vi "Scroll Home.vi"(8 "error in":errorcluster, 10 "Tab Control":T1(ring), 11 "Report Viewer in":refnum<class "Report Viewer.lvclass">) -> (0 "error out":errorcluster, 3 "Report Viewer out":refnum<class "Report Viewer.lvclass">)   [LabVIEW 2019, in "Report Viewer.lvlib" / "Report Viewer.lvclass"]
uses:
  Library/Report Viewer.lvclass
  Library/Report Viewer.lvclass/Report Viewer.ctl
  <vilib>/Utility/miscctls.llb/LVRowAndColumnUnsignedTypeDef.ctl
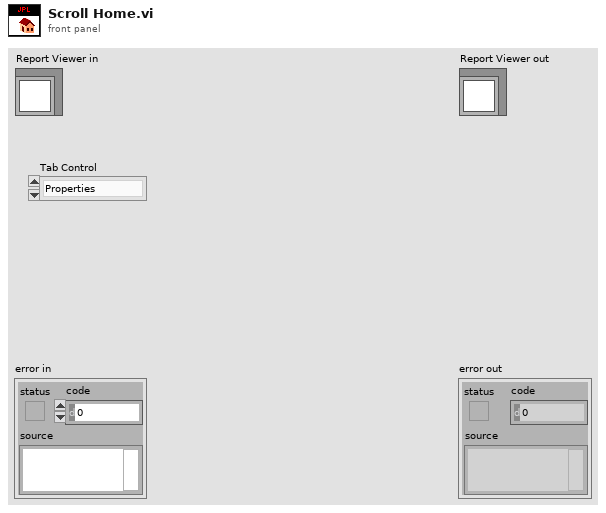
[diagram p1: front panel]
types:
  T1 = enum32{"Properties", "Values (table)", "Analog Values (Graph)"}
  T2 = enum8{"Enabled", "Disabled", "Disabled and Grayed Out"}
  T3 = typedef "LVRowAndColumnUnsignedTypeDef.ctl" = cluster{"Row":u32, "Column":u32}
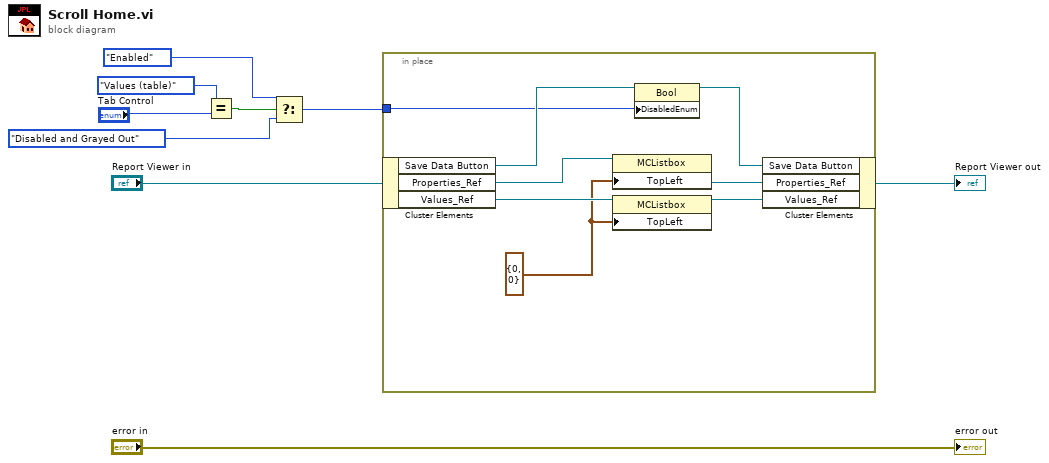
[diagram p0: block diagram]
diagram:
  n1 = Equal?(x=T1."Values (table)", y="Tab Control") -> (x = y?=w4:bool)
  n2 = Select(t=T2."Enabled" ("Disabled"), s=w4, f=T2."Disabled and Grayed Out" ("Disabled")) -> (s? t:f=w1:T2)
  n3 = in-place {
    in-place-border: w1 -> [w10]
    w13 = T3 {"Row"=0, "Column"=0} ("Top Left Visible Cell")
    n4 = in-place-cluster #1("Report Viewer in") -> ("Save Data Button"=w12:refnum<vi>, "Properties_Ref"=w15:refnum<vi>, "Values_Ref"=w17:refnum<vi>)
    n5 = property class="MCListbox"(reference=w15, "TopLeft"=w13) -> (reference out=w14:refnum<vi>)  [unwired: 1 in, 1 out]
    n6 = property class="MCListbox"(reference=w17, "TopLeft"=w13) -> (reference out=w16:refnum<vi>)  [unwired: 1 in, 1 out]
    n7 = property class="Bool"(reference=w12, "DisabledEnum"=w10) -> (reference out=w11:refnum<vi>)  [unwired: 1 in, 1 out]
    n8 = in-place-cluster #1("Save Data Button"=w11, "Properties_Ref"=w14, "Values_Ref"=w16) -> (→"Report Viewer out":refnum<class "Report Viewer.lvclass">)
  }
  "error out" <- "error in"
